vi "DUAL GAUGE-RW Filter time.vi"(7 "W/R":bool, 8 "Fehler (Eingang)":errorcluster, 9 "Sensor 2 Set":i8(ring)=1 items=["fast", "normal", "slow"], 10 "Sensor 1 Set":i8(ring)=1 items=["fast", "normal", "slow"], 11 "Referenz in":refnum<visa-resource-name>) -> (0 "Cluster (Ausgang)":errorcluster, 1 "Sensor 2 Get":i8(ring)=1 items=["fast", "normal", "slow"], 2 "Sensor 1 Get":i8(ring)=1 items=["fast", "normal", "slow"], 3 "Referenz out":refnum<visa-resource-name>)   [LabVIEW 2010, in "Dual Gauge.lvlib"]
uses:
  Dual Gauge.lvlib
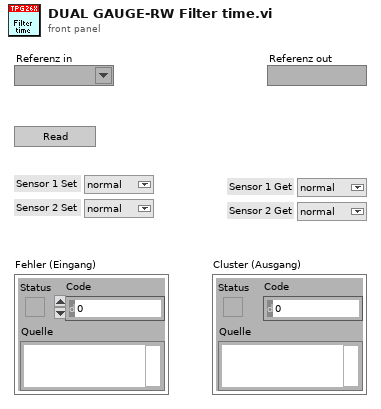
[diagram p1: front panel]
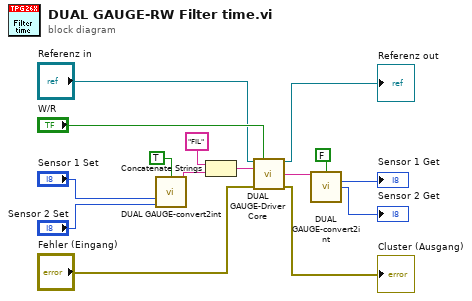
[diagram p0: block diagram]
diagram:
  n1 = call "DUAL GAUGE-convert2int.vi"("W/R [W: Int in; Str out ]"=TRUE, "Integer1 in"="Sensor 1 Set", "Integer2 in"="Sensor 2 Set") -> ("String out"=w10:string)  [unwired: 8 in, 4 out]
  n2 = Concatenate Strings("FIL", w10) -> (w7:string)
  n3 = call "DUAL GAUGE-Driver Core.vi"("Referenz in"="Referenz in", "Write/Read"="W/R", "Command"=w7, "Fehler (Eingang)"="Fehler (Eingang)") -> ("Referenz out"=→"Referenz out":refnum<visa-resource-name>, "String Out"=w8:string, "Cluster (Ausgang)"=→"Cluster (Ausgang)":errorcluster)  [unwired: 9 in]
  n4 = call "DUAL GAUGE-convert2int.vi"("String in"=w8, "W/R [W: Int in; Str out ]"=FALSE) -> ("Integer1 out"=→"Sensor 1 Get":u8, "Integer2 out"=→"Sensor 2 Get":u8)  [unwired: 9 in, 3 out]
